vi "enc to cm.vi"(0 "E":i32) -> (2 "CM":dbl)   [LabVIEW 2013]
uses:
  Global 1.vi
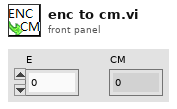
[diagram p1: front panel]
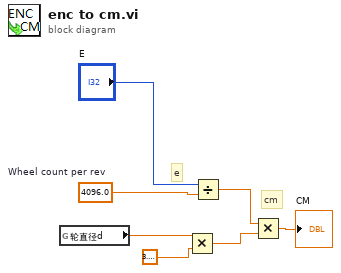
[diagram p0: block diagram]
diagram:
  w2 = 4096.0  # Wheel count per rev
  # "e"
  # "cm"
  n1 = global read "Global 1.vi" "轮直径d"() -> (w1:dbl)
  n2 = Multiply(x=w1, y=3.141592653589793) -> (x*y=w3:dbl)
  n3 = Divide(x="E", y=w2) -> (x/y=w7:dbl)
  n4 = Multiply(x=w7, y=w3) -> (x*y=→"CM":dbl)
